vi "TreeParser.vi"(0 "Tree ref in":refnum<vi>, 11 "error in (no error)":errorcluster) -> (4 "Tree Ref out":refnum<vi>, 6 "Script Array":string[](array[string]), 8 "Conditional Array out":bool[](array[boolean]), 10 "Attended? Array":bool[](array[boolean]), 15 "error out":errorcluster)   [LabVIEW 2010]
doc: "This VI parses the tree and creates a \"logical\" test sequence (Script Array)"
uses:
  Procedure_cluster.ctl
panel:
  out "Script cluster":T1[](array[typedef])
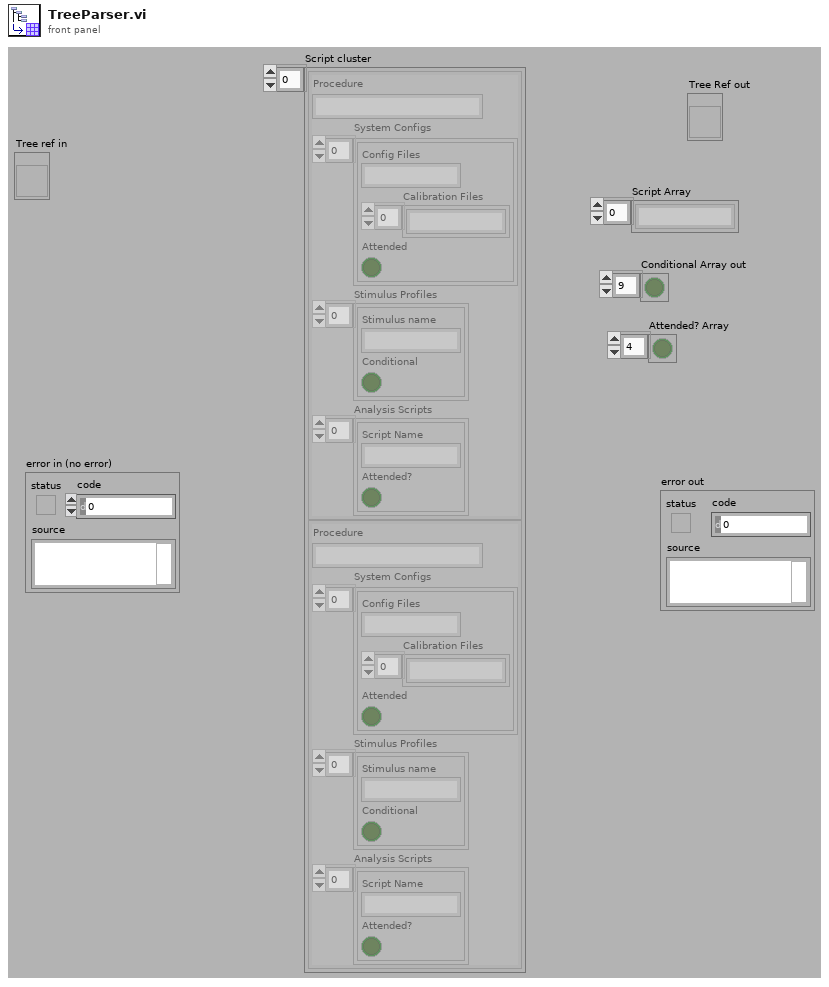
[diagram p1: front panel]
types:
  T1 = typedef "Procedure_cluster.ctl" = cluster{"Procedure":string, "System Configs":cluster{"Config Files":string, "Calibration Files":string[], "Attended":bool}[], "Stimulus Profiles":cluster{"Stimulus name":string, "Conditional":bool}[], "Analysis Scripts":cluster{"Script Name":string, "Attended?":bool}[]}
  T2 = cluster{"Config Files":string, "Calibration Files":string[], "Attended":bool}
  T3 = cluster{"Stimulus name":string, "Conditional":bool}
  T4 = cluster{"Config Files":string, "Calibration Files":string[], "Attended":bool}[]
  T5 = cluster{"Stimulus name":string, "Conditional":bool}[]
  T6 = cluster{"Script Name":string, "Attended?":bool}[]
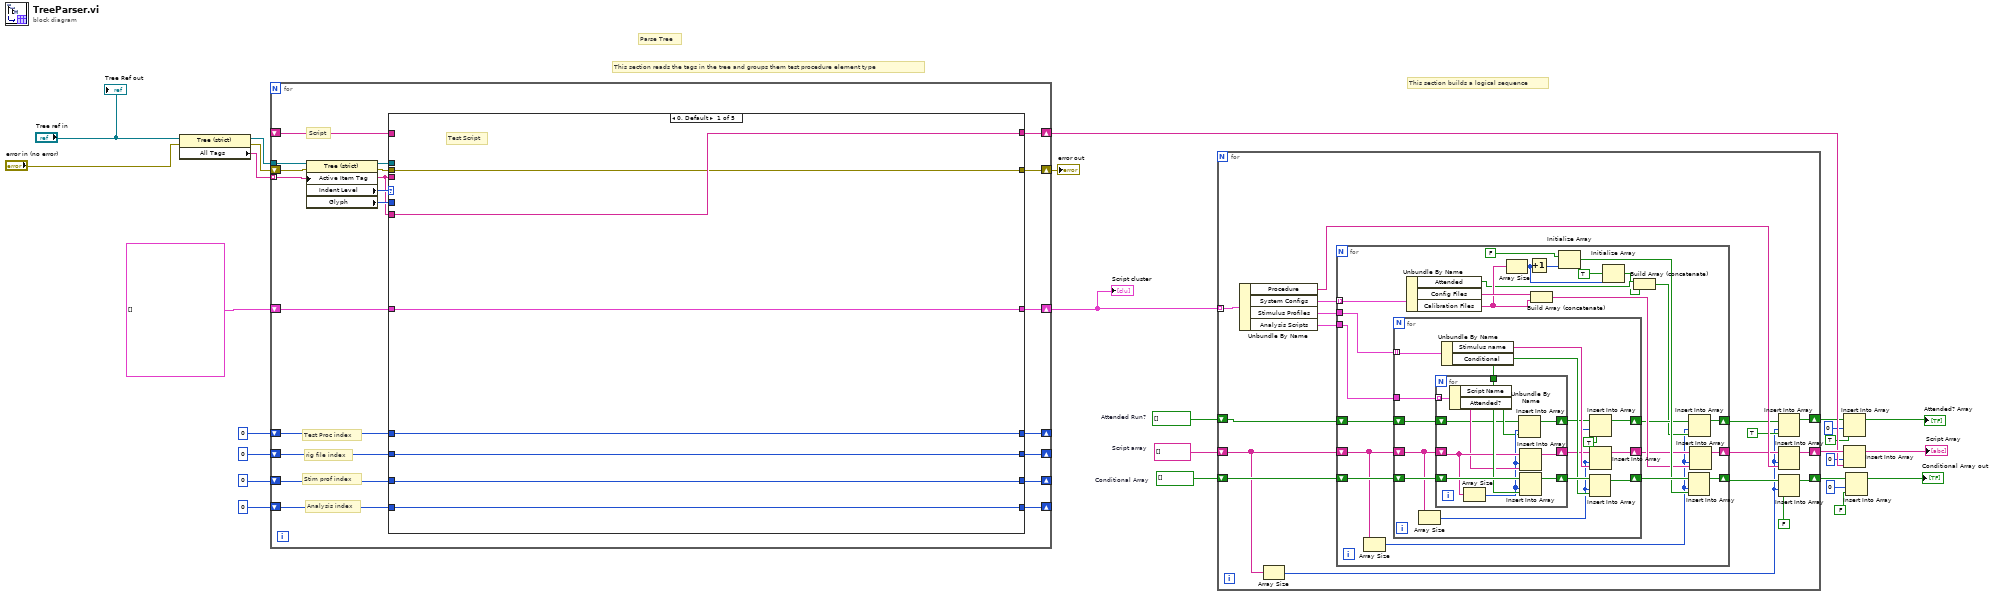
[diagram p0: block diagram]
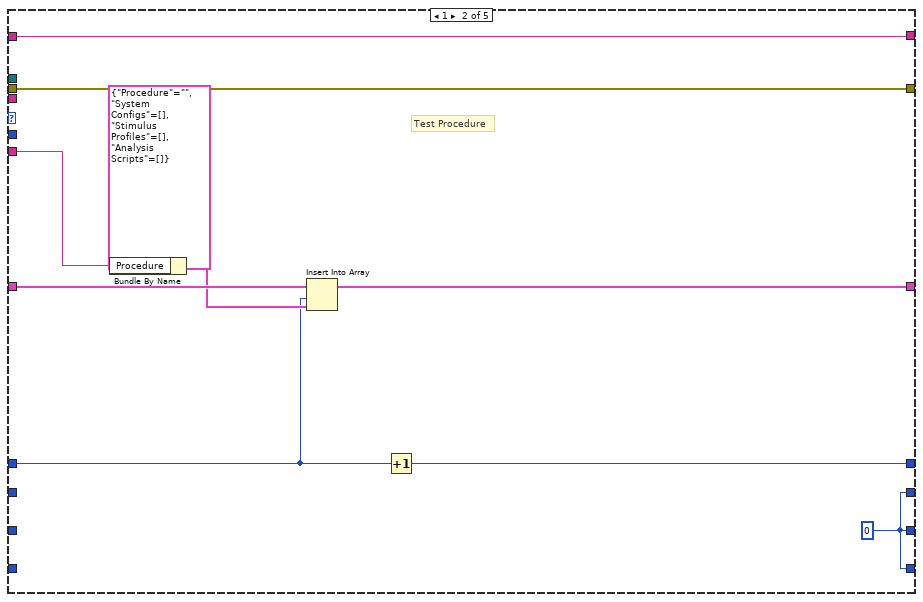
[diagram p2: hidden frame]
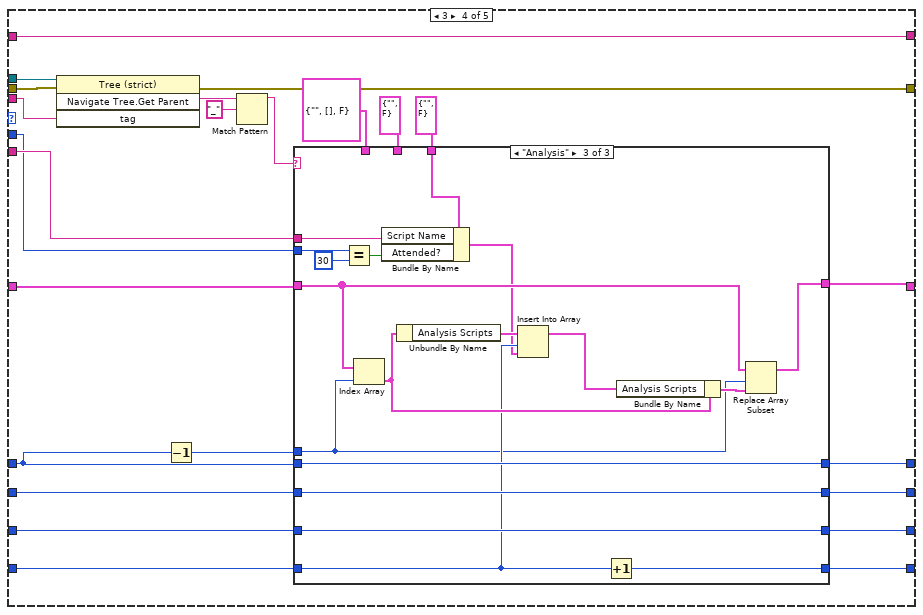
[diagram p4: hidden frame]
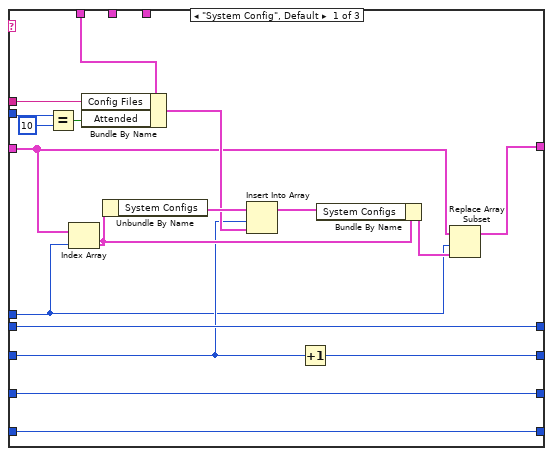
[diagram p5: hidden frame]
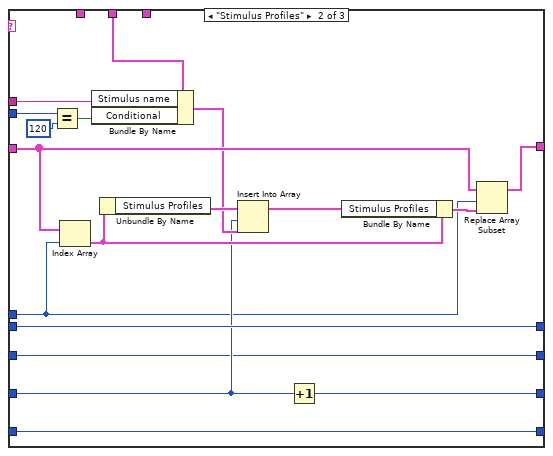
[diagram p6: hidden frame]
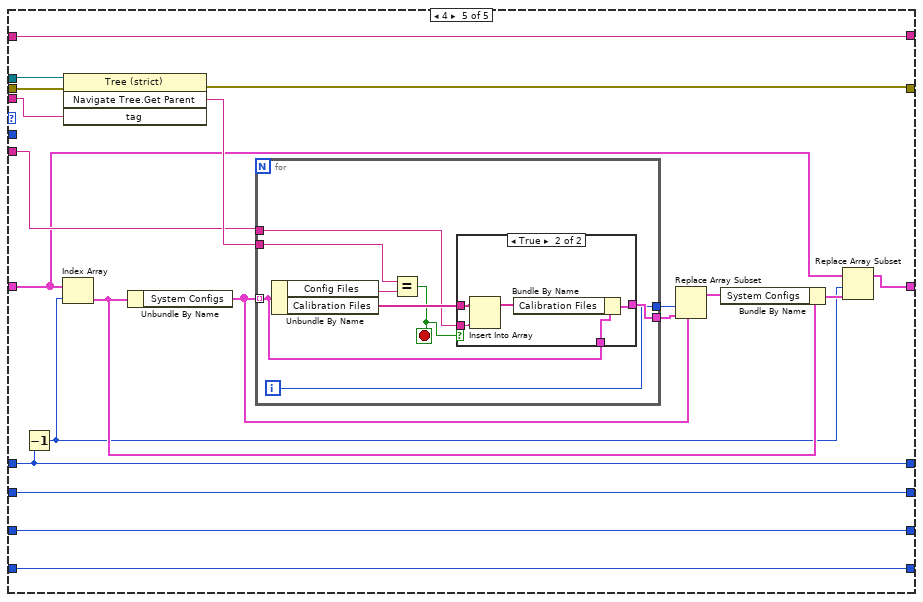
[diagram p7: hidden frame]
diagram:
  w5 = bool[] []  # Attended Run?
  w16 = bool[] []  # Conditional Array
  w23 = string[] []  # Script array
  # "This section builds a logical sequence"
  # "This section reads the tags in the tree and groups them test procedure element type"
  # "Parse Tree"
  n1 = property class="Tree (strict)"(reference="Tree ref in", error in="error in (no error)") -> (reference out=w19:refnum<vi>, error out=w25:errorcluster, "All Tags"=w18:string[])
  n2 = for {
    tunnel: w18 -> [w28] mode=indexing
    tunnel: w19 -> [w47]
    shift-right: [w43] -> w10
    shift-left: T1[] [] ("Script 2") -> [w44]
    shift-right: [w41] -> _
    shift-left: 0 -> [w42]
    shift-right: [w40] -> w22
    shift-left: _ -> [w39]
    shift-right: [w36] -> w26
    shift-left: w25 -> [w38]
    shift-right: [w33] -> _
    shift-left: 0 -> [w34]
    shift-right: [w31] -> _
    shift-left: 0 -> [w32]
    shift-right: [w29] -> _
    shift-left: 0 -> [w30]
    # "Analysis index"
    # "rig file index"
    # "Stim prof index"
    # "Script"
    # "Test Proc index"
    n3 = property class="Tree (strict)"(reference=w47, error in=w38, "Active Item Tag"=w28) -> (reference out=w45:refnum<vi>, error out=w37:errorcluster, "Indent Level"=w46:i32, "Glyph"=w35:i32)
    n4 = case shown="0, Default" w46 {
      tunnel: w28 -> [w52 w64 _ w92 w167]
      tunnel: w45 -> [_ _ _ w95 w169]
      tunnel: w44 -> [w54 w63 w71 w90 w162]
      tunnel: [w54 w61 w71 w88 w160] -> w43
      tunnel: w42 -> [w53 w56 w70 w73 w151]
      tunnel: [w53 w55 w70 w89 w151] -> w41
      tunnel: [w52 w59 w69 w87 w158] -> w40
      tunnel: w39 -> [_ w59 w69 w87 w158]
      tunnel: w37 -> [w51 w58 w68 w86 w157]
      tunnel: [w51 w58 w68 w85 w156] -> w36
      tunnel: w35 -> [_ _ _ w76 _]
      tunnel: w34 -> [w50 _ w67 w83 w155]
      tunnel: [w50 w57 w67 w82 w155] -> w33
      tunnel: w32 -> [w48 _ w66 w81 w154]
      tunnel: [w48 w57 w66 w80 w154] -> w31
      tunnel: w30 -> [w49 _ w65 w79 w153]
      tunnel: [w49 w57 w65 w78 w153] -> w29
      tunnel: w28 -> [_ _ _ w77 w152]
      frame 0, Default {
        # "Test Script"
      }
      frame 1 {
        w57 = 0
        # "Test Procedure"
        n5 = Bundle By Name(cluster=T1 {"Procedure"="", "System Configs"=[], "Stimulus Profiles"=[], "Analysis Scripts"=[]} ("Test Procedure"), "Procedure"=w64) -> (w60:T1)
        n6 = Insert Into Array(array=w63, index=w56, new element=w60) -> (w61:T1[])
        n7 = Increment(x=w56) -> (x+1=w55:i32)
      }
      frame 2 {
      }
      frame 3 {
        n8 = invoke class="Tree (strict)" method="Navigate Tree.Get Parent"(reference=w95, error in=w86, "tag"=w77) -> (error out=w85:errorcluster, "Navigate Tree:Get Parent"=w94:string)  [unwired: 1 in, 2 out]
        n9 = Decrement(x=w73) -> (x-1=w72:i32)
        n10 = Match Pattern(string=w94, regular expression="_") -> (before substring=w91:string)  [unwired: 1 in, 3 out]
        n11 = case shown="\"Analysis\"" w91 {
          tunnel: w92 -> [w111 w123 w137]
          tunnel: w90 -> [w107 w129 w147]
          tunnel: w72 -> [w96 w114 w133]
          tunnel: w73 -> [w105 w127 w145]
          tunnel: [w105 w127 w145] -> w89
          tunnel: T2 {"Config Files"="", "Calibration Files"=[], "Attended"=FALSE} ("Model Config") -> [w112 _ _]
          tunnel: [w108 w130 w148] -> w88
          tunnel: T3 {"Stimulus name"="", "Conditional"=FALSE} ("Stimulus Profile") -> [_ w124 _]
          tunnel: w83 -> [w104 w121 w143]
          tunnel: [w104 w120 w143] -> w82
          tunnel: w81 -> [w102 w119 w142]
          tunnel: [w101 w119 w142] -> w80
          tunnel: w79 -> [w100 w118 w141]
          tunnel: [w100 w118 w140] -> w78
          tunnel: w76 -> [w98 w117 w135]
          tunnel: cluster{"Script Name":string, "Attended?":bool} {"Script Name"="", "Attended?"=FALSE} ("Analysis Scripts") -> [_ _ w139]
          frame "System Config", Default {
            n12 = Equal?(x=w98, y=10) -> (x = y?=w99:bool)
            n13 = Index Array(array=w107, index=w96) -> (element=w109:T1)
            n14 = Bundle By Name(cluster=w112, "Config Files"=w111, "Attended"=w99) -> (w110:T2)
            n15 = Unbundle By Name(w109) -> ("System Configs"=w113:T4)
            n16 = Insert Into Array(array=w113, index=w102, new element=w110) -> (w103:T4)
            n17 = Increment(x=w102) -> (x+1=w101:i32)
            n18 = Bundle By Name(cluster=w109, "System Configs"=w103) -> (w106:T1)
            n19 = Replace Array Subset(array=w107, new element=w106, index=w96) -> (w108:T1[])
          }
          frame "Stimulus Profiles" {
            n20 = Equal?(x=w117, y=120) -> (x = y?=w115:bool)
            n21 = Index Array(array=w129, index=w114) -> (element=w131:T1)
            n22 = Bundle By Name(cluster=w124, "Stimulus name"=w123, "Conditional"=w115) -> (w122:T3)
            n23 = Unbundle By Name(w131) -> ("Stimulus Profiles"=w126:T5)
            n24 = Insert Into Array(array=w126, index=w121, new element=w122) -> (w125:T5)
            n25 = Increment(x=w121) -> (x+1=w120:i32)
            n26 = Bundle By Name(cluster=w131, "Stimulus Profiles"=w125) -> (w128:T1)
            n27 = Replace Array Subset(array=w129, new element=w128, index=w114) -> (w130:T1[])
          }
          frame "Analysis" {
            n28 = Equal?(x=w135, y=30) -> (x = y?=w136:bool)
            n29 = Index Array(array=w147, index=w133) -> (element=w149:T1)
            n30 = Bundle By Name(cluster=w139, "Script Name"=w137, "Attended?"=w136) -> (w138:cluster{"Script Name":string, "Attended?":bool})
            n31 = Unbundle By Name(w149) -> ("Analysis Scripts"=w144:T6)
            n32 = Insert Into Array(array=w144, index=w141, new element=w138) -> (w132:T6)
            n33 = Increment(x=w141) -> (x+1=w140:i32)
            n34 = Bundle By Name(cluster=w149, "Analysis Scripts"=w132) -> (w146:T1)
            n35 = Replace Array Subset(array=w147, new element=w146, index=w133) -> (w148:T1[])
          }
        }
      }
      frame 4 {
        n36 = Decrement(x=w151) -> (x-1=w150:i32)
        n37 = Index Array(array=w162, index=w150) -> (element=w164:T1)
        n38 = invoke class="Tree (strict)" method="Navigate Tree.Get Parent"(reference=w169, error in=w157, "tag"=w152) -> (error out=w156:errorcluster, "Navigate Tree:Get Parent"=w168:string)  [unwired: 1 in, 2 out]
        n39 = Unbundle By Name(w164) -> ("System Configs"=w166:T4)
        n40 = for {
          tunnel: w166 -> [w173] mode=indexing
          tunnel: w168 -> [w176]
          tunnel: w167 -> [w174]
          tunnel: [w172] -> w165
          tunnel: [w170] -> w159
          i -> [w170]
          stop <- w171 stop-if-true
          n41 = Unbundle By Name(w173) -> ("Config Files"=w177:string, "Calibration Files"=w175:string[])
          n42 = Equal?(x=w176, y=w177) -> (x = y?=w171:bool)
          n43 = case shown="True" w171 {
            tunnel: w175 -> [_ w183]
            tunnel: w174 -> [_ w182]
            tunnel: w173 -> [w178 w181]
            tunnel: [w178 w180] -> w172
            frame False {
            }
            frame True {
              n44 = Insert Into Array(array=w183, new element=w182) -> (w179:string[])  [unwired: 1 in]
              n45 = Bundle By Name(cluster=w181, "Calibration Files"=w179) -> (w180:T2)
            }
          }
        }
        n46 = Replace Array Subset(array=w166, new element=w165, index=w159) -> (w163:T4)
        n47 = Bundle By Name(cluster=w164, "System Configs"=w163) -> (w161:T1)
        n48 = Replace Array Subset(array=w162, new element=w161, index=w150) -> (w160:T1[])
      }
    }
  }
  "Script cluster" <- w10
  "error out" <- w26
  n49 = for {
    tunnel: w10 -> [w200] mode=indexing
    shift-right: [w194] -> w24
    shift-left: w23 -> [w185]
    shift-right: [w192] -> w15
    shift-left: w16 -> [w195]
    shift-right: [w187] -> w4
    shift-left: w5 -> [w190]
    n50 = Unbundle By Name(w200) -> ("Procedure"=w196:string, "System Configs"=w199:T4, "Stimulus Profiles"=w198:T5, "Analysis Scripts"=w197:T6)
    n51 = Array Size(array=w185) -> (size(s)=w184:i32)
    n52 = for {
      tunnel: w199 -> [w224] mode=indexing
      tunnel: w198 -> [w223]
      tunnel: w197 -> [w222]
      shift-right: [w221] -> w186
      shift-left: w185 -> [w202]
      shift-right: [w217] -> w193
      shift-left: w195 -> [w219]
      shift-right: [w209] -> w189
      shift-left: w190 -> [w211]
      n53 = Array Size(array=w202) -> (size(s)=w201:i32)
      n54 = for {
        tunnel: w223 -> [w238] mode=indexing
        tunnel: w222 -> [w239]
        shift-right: [w231] -> w203
        shift-left: w202 -> [w226]
        shift-right: [w234] -> w218
        shift-left: w219 -> [w236]
        shift-right: [w230] -> w210
        shift-left: w211 -> [w232]
        n55 = Array Size(array=w226) -> (size(s)=w225:i32)
        n56 = Unbundle By Name(w238) -> ("Stimulus name"=w237:string, "Conditional"=w233:bool)
        n57 = for {
          tunnel: w239 -> [w250] mode=indexing
          shift-right: [w249] -> w227
          shift-left: w226 -> [w245]
          shift-right: [w246] -> w235
          shift-left: w236 -> [w248]
          tunnel: w233 -> [w247]
          shift-right: [w240] -> w229
          shift-left: w232 -> [w241]
          n58 = Unbundle By Name(w250) -> ("Script Name"=w244:string, "Attended?"=w242:bool)
          n59 = Array Size(array=w245) -> (size(s)=w243:i32)
          n60 = Insert Into Array(array=w241, index=w243, new element=w242) -> (w240:bool[])
          n61 = Insert Into Array(array=w245, index=w243, new element=w244) -> (w249:string[])
          n62 = Insert Into Array(array=w248, index=w243, new element=w247) -> (w246:bool[])
        }
        n63 = Insert Into Array(array=w235, index=w225, new element=w233) -> (w234:bool[])
        n64 = Insert Into Array(array=w229, index=w225, new element=TRUE ("new element/subarray")) -> (w230:bool[])
        n65 = Insert Into Array(array=w227, index=w225, new element=w237) -> (w231:string[])
      }
      n66 = Unbundle By Name(w224) -> ("Attended"=w206:bool, "Config Files"=w220:string, "Calibration Files"=w216:string[])
      n67 = Array Size(array=w216) -> (size(s)=w207:i32)
      n68 = Increment(x=w207) -> (x+1=w215:i32)
      n69 = Build Array (concatenate)(w220, w216) -> (w212:string[])
      n70 = Initialize Array(FALSE ("new element/subarray"), w215) -> (w213:bool[])
      n71 = Initialize Array(TRUE ("element"), w207) -> (w205:bool[])
      n72 = Build Array (concatenate)(w206, w205) -> (w204:bool[])
      n73 = Insert Into Array(array=w218, index=w201, new element=w213) -> (w217:bool[])
      n74 = Insert Into Array(array=w210, index=w201, new element=w204) -> (w209:bool[])
      n75 = Insert Into Array(array=w203, index=w201, new element=w212) -> (w221:string[])
    }
    n76 = Insert Into Array(array=w189, index=w184, new element=TRUE ("new element/subarray")) -> (w187:bool[])
    n77 = Insert Into Array(array=w186, index=w184, new element=w196) -> (w194:string[])
    n78 = Insert Into Array(array=w193, index=w184, new element=FALSE ("new element/subarray")) -> (w192:bool[])
  }
  n79 = Insert Into Array(array=w4, index=0, new element=TRUE ("new element/subarray")) -> (→"Attended? Array":bool[])
  n80 = Insert Into Array(array=w24, index=0, new element=w22) -> (→"Script Array":string[])
  n81 = Insert Into Array(array=w15, index=0, new element=FALSE ("new element/subarray")) -> (→"Conditional Array out":bool[])
  "Tree Ref out" <- "Tree ref in"
